vi "MUX80_Split_Page_Double.vi"(0 "Array In":dbl[](array[numeric]) format="%.6f") -> (1 "Page 1 out":dbl[](array[numeric]) format="%.6f", 2 "Page 6 out":dbl[](array[numeric]) format="%.6f", 3 "Page 2 out":dbl[](array[numeric]) format="%.6f", 4 "Page 3 out":dbl[](array[numeric]) format="%.6f", 5 "Page 4 out":dbl[](array[numeric]) format="%.6f", 6 "Page 5 out":dbl[](array[numeric]) format="%.6f")   [LabVIEW 2020]
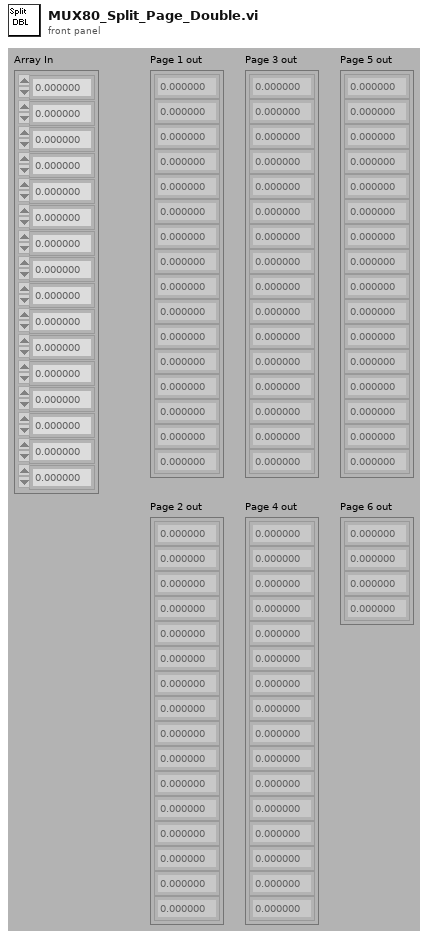
[diagram p1: front panel]
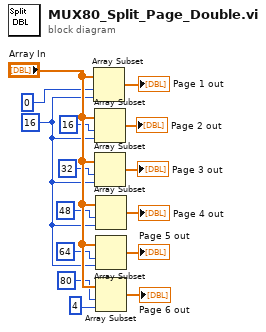
[diagram p0: block diagram]
diagram:
  w7 = 16
  n1 = Array Subset(array="Array In", index=0, length=w7) -> (→"Page 1 out":dbl[])
  n2 = Array Subset(array="Array In", index=16, length=w7) -> (→"Page 2 out":dbl[])
  n3 = Array Subset(array="Array In", index=32, length=w7) -> (→"Page 3 out":dbl[])
  n4 = Array Subset(array="Array In", index=48, length=w7) -> (→"Page 4 out":dbl[])
  n5 = Array Subset(array="Array In", index=64, length=w7) -> (→"Page 5 out":dbl[])
  n6 = Array Subset(array="Array In", index=80, length=4) -> (→"Page 6 out":dbl[])
